vi "UHR-Fleezers Control (host) -TL - oscillation.vi"(0 "Tab Control":T5(tab)) -> ()   [LabVIEW 2013] (continued)
    n1506 = Split 1D Array(array=w2057, index="N El. to Ave.") -> (second subarray=w2060:dbl[])  [unwired: 1 out]
    n1507 = Split 1D Array(array=w2054, index="N El. to Ave.") -> (second subarray=w2059:dbl[])  [unwired: 1 out]
    n1508 = local read "Trap X AI1 (DMA)"() -> (w2058:T13)
    n1509 = Multiply(x=w2132, y="Trap Disp. Downsample") -> (x*y=w2071:dbl)
    "Display Period (s)" <- w2071
    n1510 = Bundle("BD 1 Frequency 1 (MHz)"=w2026, "BD 1 Frequency 2 (MHz)"=w2025) -> (w2027:T45)  [unwired: 1 out]
    n1511 = for "Trap AI" {
      tunnel: [w2677] -> w2257 mode=indexing
      tunnel: w2069 -> [w2667]
      tunnel: "Trap Disp. Downsample" -> [w2675]
      tunnel: w2150 -> [w2673] mode=indexing
      tunnel: w2132 -> [w2672]
      tunnel: w2149 -> [w2671] mode=indexing
      tunnel: w2068 -> [w2670]
      tunnel: [w2669] -> w2107 mode=indexing
      tunnel: w2071 -> [w2668]
      n1512 = Bundle By Name("Y"=w2673, "dt"=w2672) -> (w2674:waveform(dbl))  [unwired: 1 out]
      n1513 = Set Waveform Attribute(5:w2671, 6:w2670, 7:w2674) -> (3:w2669:waveform(dbl))  [unwired: 1 in, 2 out]
      n1514 = call "downsample 1D array - double.vi"("Ave N"=w2675, "Array In"=w2673) -> ("Array Out"=w2676:dbl[])  [unwired: 1 out]
      n1515 = Bundle By Name(cluster=w2669, "t0"=w2667, "Y"=w2676, "dt"=w2668) -> (w2677:waveform(dbl))
    }
    n1516 = call-poly <vilib>:"Mean.vi"("X"=w2059) -> ("mean"=w2047:dbl)  [unwired: 1 out]
    n1517 = call-poly <vilib>:"Mean.vi"("X"=w2060) -> ("mean"=w2048:dbl)  [unwired: 1 out]
    n1518 = Cluster To Array(cluster=w2027) -> (array=w2024:dbl[])
    n1519 = Reciprocal(x=w2071) -> (1/x=→"Trap Disp. Freq. (Hz)":dbl)
    n1520 = local read "Data points/scans (MCL)"() -> (w2237:dbl)
    n1521 = To Fixed-Point(number=w2047) -> (fixed-point=w2045:fxp<+/-,16,1>)  [unwired: 1 in]
    n1522 = To Fixed-Point(number=w2048) -> (fixed-point=w2046:fxp<+/-,16,1>)  [unwired: 1 in]
    n1523 = Bundle("Trap 1 Pos.", "Trap 2 Pos.") -> (w2067:cluster{string, string})  [unwired: 1 out]
    n1524 = Bundle By Name(cluster=w2058, "Set 1"=w2046, "Set 2"=w2045) -> (→"Trap X AI1 (DMA)":T13)
    n1525 = Cluster To Array(cluster=w2067) -> (array=w2064:string[])
    n1526 = for "Trap Position" {
      tunnel: w2073 -> [w2317] mode=indexing
      tunnel: "Trap Disp. Downsample" -> [w2316]
      tunnel: w2071 -> [w2314]
      tunnel: w2069 -> [w2313]
      tunnel: w2068 -> [w2311]
      tunnel: w2064 -> [w2310] mode=indexing
      tunnel: [w2309] -> w2022 mode=indexing
      tunnel: w2024 -> [w2307] mode=indexing
      tunnel: w2023 -> [w2305]
      n1527 = call "downsample 1D array - double.vi"("Ave N"=w2316, "Array In"=w2317) -> ("Array Out"=w2315:dbl[])  [unwired: 1 out]
      n1528 = Subtract(x=w2315, y=w2307) -> (x-y=w2308:dbl[])
      n1529 = Multiply(x=w2305, y=w2308) -> (x*y=w2306:dbl[])
      n1530 = Bundle By Name("Y"=w2306, "dt"=w2314, "t0"=w2313) -> (w2312:waveform(dbl))  [unwired: 1 out]
      n1531 = Set Waveform Attribute(5:w2310, 6:w2311, 7:w2312) -> (3:w2309:waveform(dbl))  [unwired: 1 in, 2 out]
    }
    "Trap Positions" <- w2022
    n1532 = Bundle("APD 1", "APD 2") -> (w2256:cluster{string, string})  [unwired: 1 out]
    n1533 = Cluster To Array(cluster=w2256) -> (array=w2253:string[])
    n1534 = for "APD" {
      tunnel: w2226 -> [w2656] mode=indexing
      tunnel: w2096 -> [w2664]
      tunnel: [w2660] -> w2103 mode=indexing
      tunnel: "APD Disp. Scale" -> [w2661]
      tunnel: w2068 -> [w2659]
      tunnel: w2253 -> [w2658] mode=indexing
      tunnel: "APD Disp. Downsample" -> [w2654]
      tunnel: [w2657] -> w2252
      tunnel: w2069 -> [w2653]
      n1535 = call "integrate 1D array interval - double.vi"("Ave N"=w2654, "Array In"=w2656) -> ("Array Out"=w2655:dbl[])  [unwired: 1 out]
      n1536 = Multiply(x=w2664, y=w2654) -> (x*y=w2657:dbl)
      n1537 = Divide(x=w2655, y=w2661) -> (x/y=w2662:dbl[])
      n1538 = Bundle By Name("t0"=w2653, "Y"=w2662, "dt"=w2657) -> (w2663:waveform(dbl))  [unwired: 1 out]
      n1539 = Set Waveform Attribute(5:w2658, 6:w2659, 7:w2663) -> (3:w2660:waveform(dbl))  [unwired: 1 in, 2 out]
    }
    "APD Display Period (s)" <- w2252
    n1540 = Reciprocal(x=w2252) -> (1/x=→"APD Display Freq. (Hz)":dbl)
    n1541 = local read "Display Period (s)"() -> (w2131:dbl)
    n1542 = Increment(x=w2237) -> (x+1=w2238:dbl)
    n1543 = Index Array(array=w2022, index=0) -> (element=w2020:waveform(dbl))
    n1544 = To Double Precision Float(number=w2147) -> (double precision float=w2146:dbl[])
    n1545 = feedback #2(w2238) -> (w2241:dbl)
    n1546 = Select(t=0, s=w2228, f=w2241) -> (s? t:f=w2234:dbl)
    n1547 = Array Size(array=w2146) -> (size(s)=w2240:i32)
    n1548 = Add(x=w2240, y=w2234) -> (x+y=w2235:dbl)
    n1549 = Unbundle By Name(w2020) -> ("Y"=w2018:dbl[])
    n1550 = feedback #3(w2147) -> (w2224:u32[])
    n1551 = Build Array (concatenate)(w2224, w2147) -> (w2221:u32[])
    n1552 = feedback #4(w2083) -> (w2102:u32[])
    n1553 = Divide(x="Bead Sep. Int. Time (s)", y=w2131) -> (x/y=w2016:dbl)
    n1554 = Build Array (concatenate)(w2102, w2083) -> (w2101:u32[])
    n1555 = Greater?(x=w2235, y=w2237) -> (0:w2236:bool)
    n1556 = feedback #5(w2018) -> (w2019:dbl[])
    n1557 = Build Array (concatenate)(w2018, w2019) -> (w2017:dbl[])
    n1558 = Select(t=w2234, s=w2236, f=w2235) -> (s? t:f=w2233:dbl)
    n1559 = feedback-in #2(w2233) -> ()
    n1560 = Array Size(array=w2221) -> (size(s)=w2218:i32)
    n1561 = Array Size(array=w2147) -> (size(s)=w2220:i32)
    n1562 = local read "MCL Scanning"() -> (w2231:bool)
    n1563 = local read "APD Integration Time (s)"() -> (w2110:dbl)
    n1564 = Build Array (concatenate)(w2103, w2257) -> (w2105:waveform(dbl)[])
    "All Signals" <- w2105
    n1565 = Split 1D Array(array=w2017, index=w2016) -> (first subarray=w2010:dbl[])  [unwired: 1 out]
    n1566 = feedback-in #5(w2010) -> ()
    n1567 = Multiply(x=w2220, y="APD Ave N") -> (x*y=w2219:dbl)
    n1568 = Greater?(x=w2218, y=w2219) -> (0:w2222:bool)
    n1569 = Not(x=w2236) -> (.not. x?=w2230:bool)
    n1570 = To Double Precision Float(number=w2083) -> (double precision float=w2082:dbl[])
    n1571 = call-poly <vilib>:"Mean.vi"("X"=w2010) -> ("mean"=w2009:dbl)  [unwired: 1 out]
    "Mean T1 Position (nm)" <- w2009
    n1572 = Subtract(x=w2010, y=w2009) -> (x-y=w2015:dbl[])
    n1573 = Square(x=w2015) -> (x^2=w2014:dbl[])
    n1574 = And(x=w2230, y=w2231) -> (x .and. y?=w2232:bool)
    n1575 = call-poly <vilib>:"Mean.vi"("X"=w2014) -> ("mean"=w2013:dbl)  [unwired: 1 out]
    n1576 = case shown="True" w2222 {
      tunnel: w2221 -> [w2437 w2444]
      tunnel: [w2437 w2442] -> w2163
      tunnel: w2219 -> [_ w2439]
      tunnel: w2218 -> [_ w2443]
      tunnel: w2101 -> [w2436 w2441]
      tunnel: [w2436 w2438] -> w2098
      frame False {
      }
      frame True {
        n1577 = Subtract(x=w2443, y=w2439) -> (x-y=w2440:dbl)
        n1578 = Array Subset(array=w2444, index=w2440, length=w2439) -> (w2442:u32[])
        n1579 = Array Subset(array=w2441, index=w2440, length=w2439) -> (w2438:u32[])
      }
    }
    n1580 = feedback-in #3(w2163) -> ()
    n1581 = feedback-in #4(w2098) -> ()
    n1582 = Or(x=w2232, y=w2228) -> (x .or. y?=w2229:bool)
    n1583 = Square Root(x=w2013) -> (sqrt(x)=w2012:dbl)
    n1584 = Equal?(x="Tab Control 6", y=T35."High Res Display") -> (x = y?=w2153:bool)
    n1585 = Multiply(x="APD Disp. Scale", y=w2103) -> (x*y=w2112:waveform(dbl)[])
    n1586 = Multiply(x="APD Disp. Downsample", y=w2110) -> (x*y=w2108:dbl)
    n1587 = Multiply(x=10.0, y=w2012) -> (x*y=→"Trap 1 Position RMS (A)":dbl)
    n1588 = Divide(x=w2112, y=w2108) -> (x/y=w2080:waveform(dbl)[])
    n1589 = Index Array(array=w2080, index=0) -> (element=w2090:waveform(dbl))
    n1590 = case "For computing FFTs for display" shown="True" "Compute FFT" {
      tunnel: w2107 -> [_ w3114]
      frame False {
      }
      frame True {
        n1591 = Build Array("FFT 1 Choice 1", "FFT 1 Choice 2", "FFT 2 Choice 1", "FFT 2 Choice 2") -> (w3107:u16[])
        n1592 = Array Size(array=w3114) -> (size(s)=w3113:i32)
        n1593 = feedback-in #6(w3107) -> ()
        n1594 = feedback #6(u16[] [100, 100, 100, 100]) -> (w3108:u16[])
        n1595 = feedback-in #7("# Spectra to Ave.") -> ()
        n1596 = feedback #7("# Spectra to Ave.") -> (w3105:dbl)
        n1597 = Not Equal?(x="# Spectra to Ave.", y=w3105) -> (x != y?=w3104:bool)
        n1598 = Not Equal?(x=w3107, y=w3108) -> (x != y?=w3106:bool)
        n1599 = feedback #8(1.0) -> (w3091:dbl)
        n1600 = Compound Arithmetic op=OR("Reset FFT", w3106, w3104) -> (w3089:bool)
        n1601 = Select(t=1.0, s=w3089, f=w3091) -> (s? t:f=w3093:dbl)
        n1602 = Greater?(x=w3093, y="# Spectra to Ave.") -> (0:w3112:bool)
        n1603 = Increment(x=w3093) -> (x+1=w3092:dbl)
        n1604 = feedback-in #8(w3092) -> ()
        n1605 = local read "DMA Update Period (s)"() -> (w3087:dbl)
        n1606 = Multiply(x="# Spectra to Ave.", y=w3087) -> (x*y=→"Ave. Time (s)":dbl)
        n1607 = Build Array(cluster{"f0":dbl, "df":dbl, "magnitude":dbl[]} {"f0"=0.0, "df"=0.0, "magnitude"=[]} ("PSD")) -> (w3096:cluster{"f0":dbl, "df":dbl, "magnitude":dbl[]}[])
        n1608 = Build Array(w3096, w3096, w3096, w3096) -> (w3098:T46)
        n1609 = feedback #9(w3098) -> (w3103:T46)
        n1610 = for {
          N: 4 -> [_]
          tunnel: w3107 -> [w3136] mode=indexing
          tunnel: w3114 -> [w3137]
          tunnel: w3113 -> [w3139]
          tunnel: w3089 -> [w3132]
          tunnel: w3112 -> [w3131]
          tunnel: "# Spectra to Ave." -> [w3130]
          tunnel: [w3129] -> w3102 mode=indexing
          tunnel: w3103 -> [w3134] mode=indexing
          tunnel: [w3133] -> w3090 mode=indexing
          tunnel: w3093 -> [w3128]
          n1611 = Less?(x=w3136, y=w3139) -> (x < y?=w3138:bool)
          n1612 = Index Array(array=w3137, index=w3136) -> (element=w3135:waveform(dbl))
          n1613 = case shown="True" w3138 {
            tunnel: w3135 -> [_ w3156]
            tunnel: w3134 -> [w3141 w3154]
            tunnel: [w3141 w3142] -> w3133
            tunnel: w3132 -> [_ w3153]
            tunnel: w3131 -> [_ w3146]
            tunnel: w3130 -> [_ w3145]
            tunnel: [cluster{"f0":dbl, "df":dbl, "magnitude":dbl[]} {"f0"=0.0, "df"=0.0, "magnitude"=[]} ("PSD") w3147] -> w3129
            tunnel: w3128 -> [_ w3144]
            frame False {
            }
            frame True {
              n1614 = call <vilib>:"Std Deviation and Variance.vi"("X"=w3156) -> ("mean"=w3157:dbl)  [unwired: 1 in, 2 out]
              n1615 = Subtract(x=w3156, y=w3157) -> (x-y=w3155:waveform(dbl))
              n1616 = xnode "Spectral Measurements"("Signals"=w3155) -> ("PSD"=w3149:cluster{"f0":dbl, "df":dbl, "magnitude":dbl[]})  [unwired: 1 in, 1 out]
              n1617 = case shown="False" w3153 {
                tunnel: w3154 -> [w3166 _]
                tunnel: [w3162 w3171] -> w3142
                tunnel: w3149 -> [w3165 w3172]
                tunnel: w3146 -> [w3164 _]
                frame False {
                  n1618 = Build Array (concatenate)(w3166, w3165) -> (w3163:cluster{"f0":dbl, "df":dbl, "magnitude":dbl[]}[])
                  n1619 = case shown="True" w3164 {
                    tunnel: w3163 -> [w3167 w3170]
                    tunnel: [w3167 w3168] -> w3162
                    frame False {
                    }
                    frame True {
                      n1620 = Delete From Array(array=w3170, index=0) -> (array with subset deleted=w3168:cluster{"f0":dbl, "df":dbl, "magnitude":dbl[]}[])  [unwired: 1 in, 1 out]
                    }
                  }
                }
                frame True {
                  n1621 = Build Array(w3172) -> (w3171:cluster{"f0":dbl, "df":dbl, "magnitude":dbl[]}[])
                }
              }
              n1622 = for {
                tunnel: w3142 -> [w3161] mode=indexing
                tunnel: [w3160] -> w3152 mode=indexing
                workers-P: _ -> [_]
                n1623 = Unbundle By Name(w3161) -> ("magnitude"=w3160:dbl[])
              }
              n1624 = Transpose 2D Array(2D array=w3152) -> (transposed array=w3151:dbl[][])
              n1625 = for {
                tunnel: w3151 -> [w3159] mode=indexing
                tunnel: [w3158] -> w3150 mode=indexing
                workers-P: _ -> [_]
                n1626 = Add Array Elements(numeric array=w3159) -> (sum=w3158:dbl)
              }
              n1627 = Select(t=w3145, s=w3146, f=w3144) -> (s? t:f=w3143:dbl)
              n1628 = Divide(x=w3150, y=w3143) -> (x/y=w3148:dbl[])
              n1629 = Bundle By Name(cluster=w3149, "magnitude"=w3148) -> (w3147:cluster{"f0":dbl, "df":dbl, "magnitude":dbl[]})
            }
          }
        }
        n1630 = case shown="True" w3089 {
          tunnel: w3090 -> [w3121 w3127]
          tunnel: [w3121 w3122] -> w3088
          frame False {
          }
          frame True {
            n1631 = Array Subset(array=w3127, index (row)=0 ("index"), length (row)=4 ("length"), index (col)=0 ("index"), length (col)=1 ("length")) -> (w3122:T46)
          }
        }
        n1632 = feedback-in #9(w3088) -> ()
        n1633 = Split 1D Array(array=w3102, index=2) -> (first subarray=→"FFT 1":cluster{"f0":dbl, "df":dbl, "magnitude":dbl[]}[], second subarray=→"FFT 2":cluster{"f0":dbl, "df":dbl, "magnitude":dbl[]}[])
      }
    }
    n1634 = Index Array(array=w2080, index=1) -> (element=w2088:waveform(dbl))
    n1635 = case "For displaying the high resolution display (no downsampling)" shown="True" w2153 {
      tunnel: w2107 -> [_ w2337]
      frame False {
      }
      frame True {
        n1636 = Index Array(array=w2337, index="High Res. Display") -> (element=w2338:waveform(dbl))
        n1637 = call <vilib>:"Std Deviation and Variance.vi"("X"=w2338) -> ("mean"=w2345:dbl, "standard deviation"=w2350:dbl)  [unwired: 1 in, 1 out]
        "Mean Intensity" <- w2345
        "Sigma" <- w2350
        n1638 = Subtract(x=w2338, y=w2345) -> (x-y=w2344:waveform(dbl))
        n1639 = Select(t=w2344, s="Subtract mean", f=w2338) -> (s? t:f=→"1 Channel":waveform(dbl))
        n1640 = Divide(x=w2350, y=w2345) -> (x/y=→"Sigma/Mean":dbl)
        n1641 = feedback #10(1) -> (w2339:i32)
        n1642 = Greater Or Equal?(x=w2339, y="Slow mean N ave.") -> (x >= y?=w2352:bool)
        n1643 = Increment(x=w2339) -> (x+1=w2354:i32)
        n1644 = Select(t=1, s=w2352, f=w2354) -> (s? t:f=w2341:i32)
        n1645 = feedback-in #10(w2341) -> ()
        n1646 = feedback #11() -> (w2342:waveform(dbl))  [unwired: 1 out]
        n1647 = case shown="Default" w2339 {
          tunnel: [w2357 w2360] -> w2343
          tunnel: w2342 -> [w2359 _]
          tunnel: w2338 -> [w2358 w2360]
          frame Default {
            n1648 = call-poly <vilib>:"Append Waveforms.vi"("waveform B"=w2358, "waveform A"=w2359) -> ("waveform out"=w2357:waveform(dbl))  [unwired: 1 in, 8 out]
          }
          frame 1 {
          }
        }
        n1649 = feedback-in #11(w2343) -> ()
        n1650 = case shown="True" w2352 {
          tunnel: w2343 -> [_ w2356]
          frame False {
          }
          frame True {
            n1651 = call-poly <vilib>:"Mean.vi"("X"=w2356) -> ("mean"=→"Slow mean":dbl)  [unwired: 1 out]
          }
        }
      }
    }
    n1652 = case "For plotting results of scanning MCL" shown="True" w2229 {
      tunnel: w2228 -> [_ w2477]
      tunnel: w2146 -> [_ w2573]
      tunnel: w2237 -> [_ _]
      tunnel: w2107 -> [_ w2547]
      tunnel: w2082 -> [_ w2478]
      tunnel: w2081 -> [_ w2451]
      frame False {
      }
      frame True {
        w2458 = u32 0 items=["Horizontal", "Vertical", "Central", "1st Diagonal", "2nd Diagonal"] ("Type of Symmetry")
        w2486 = u32 0 items=["Horizontal", "Vertical", "Central", "1st Diagonal", "2nd Diagonal"] ("Type of Symmetry")
        w2489 = u32 0 items=["Horizontal", "Vertical", "Central", "1st Diagonal", "2nd Diagonal"] ("Type of Symmetry")
        w2518 = u32 0 items=["Horizontal", "Vertical", "Central", "1st Diagonal", "2nd Diagonal"] ("Type of Symmetry")
        n1653 = Index Array(array=w2547, index=10) -> (element=w2553:waveform(dbl))
        n1654 = Index Array(array=w2547, index=11) -> (element=w2550:waveform(dbl))
        n1655 = local read "Cycles/step (MCL)"() -> (w2503:u64)
        n1656 = Index Array(array=w2547, index="Channel") -> (element=w2549:waveform(dbl))
        n1657 = Unbundle(w2451) -> ("New Image"=w2450:T3, "New Image"=w2449:T3, "New Image"=w2448:T3, "New Image"=w2447:T3)
        n1658 = Unbundle By Name(w2553) -> ("Y"=w2505:dbl[])
        n1659 = Unbundle By Name(w2550) -> ("Y"=w2507:dbl[])
        n1660 = Unbundle By Name(w2549) -> ("Y"=w2512:dbl[])
        n1661 = call "downsample 1D array - double.vi"("Ave N"=w2503, "Array In"=w2505) -> ("Array Out"=w2504:dbl[])  [unwired: 1 out]
        n1662 = call "downsample 1D array - double.vi"("Ave N"=w2503, "Array In"=w2507) -> ("Array Out"=w2506:dbl[])  [unwired: 1 out]
        n1663 = call "downsample 1D array - double.vi"("Ave N"=w2503, "Array In"=w2512) -> ("Array Out"=w2511:dbl[])  [unwired: 1 out]
        n1664 = feedback #12(w2573) -> (w2574:dbl[])
        n1665 = Build Array (concatenate)(w2574, w2573) -> (w2555:dbl[])
        n1666 = feedback #13(w2478) -> (w2480:dbl[])
        n1667 = Build Array (concatenate)(w2480, w2478) -> (w2479:dbl[])
        n1668 = local read "Scan steps (MCL)"() -> (w2460:u64)
        n1669 = Select(t=w2573, s=w2477, f=w2555) -> (s? t:f=w2559:dbl[])
        n1670 = feedback-in #12(w2559) -> ()
        n1671 = Select(t=w2478, s=w2477, f=w2479) -> (s? t:f=w2461:dbl[])
        n1672 = feedback-in #13(w2461) -> ()
        n1673 = local read "Scan lines (y)"() -> (w2446:u64)
        n1674 = local read "N APD Samp/step"() -> (w2462:dbl)
        n1675 = feedback #14(w2504) -> (w2561:dbl[])
        n1676 = Build Array (concatenate)(w2561, w2504) -> (w2552:dbl[])
        n1677 = feedback #15(w2511) -> (w2571:dbl[])
        n1678 = Build Array (concatenate)(w2571, w2511) -> (w2570:dbl[])
        n1679 = feedback #16(w2506) -> (w2563:dbl[])
        n1680 = Build Array (concatenate)(w2563, w2506) -> (w2564:dbl[])
        n1681 = Select(t=w2504, s=w2477, f=w2552) -> (s? t:f=w2508:dbl[])
        n1682 = feedback-in #14(w2508) -> ()
        n1683 = Select(t=w2511, s=w2477, f=w2570) -> (s? t:f=w2510:dbl[])
        n1684 = feedback-in #15(w2510) -> ()
        n1685 = Select(t=w2506, s=w2477, f=w2564) -> (s? t:f=w2509:dbl[])
        n1686 = feedback-in #16(w2509) -> ()
        n1687 = Multiply(x=w2460, y=u64 2) -> (x*y=w2445:u64)
        n1688 = call "integrate 1D array interval - double.vi"("Ave N"=w2462, "Array In"=w2461) -> ("Array Out"=w2473:dbl[])  [unwired: 1 out]
        n1689 = call "integrate 1D array interval - double.vi"("Ave N"=w2462, "Array In"=w2559) -> ("Array Out"=w2558:dbl[])  [unwired: 1 out]
        n1690 = Array Size(array=w2473) -> (size(s)=w2474:i32)
        n1691 = Array Size(array=w2558) -> (size(s)=w2560:i32)
        n1692 = Multiply(x=w2446, y=w2445) -> (x*y=w2476:u64)
        n1693 = Multiply(x=w2446, y=w2445) -> (x*y=w2568:u64)
        n1694 = call-poly <vilib>:"Mean.vi"("X"=w2508) -> ("mean"=w2492:dbl)  [unwired: 1 out]
        n1695 = Subtract(x=w2476, y=w2474) -> (x-y=w2467:u64)
        n1696 = call-poly <vilib>:"Mean.vi"("X"=w2510) -> ("mean"=w2497:dbl)  [unwired: 1 out]
        n1697 = call-poly <vilib>:"Mean.vi"("X"=w2509) -> ("mean"=w2495:dbl)  [unwired: 1 out]
        n1698 = call-poly <vilib>:"Mean.vi"("X"=w2473) -> ("mean"=w2464:dbl)  [unwired: 1 out]
        n1699 = Subtract(x=w2568, y=w2560) -> (x-y=w2502:u64)
        n1700 = call-poly <vilib>:"Mean.vi"("X"=w2558) -> ("mean"=w2499:dbl)  [unwired: 1 out]
        n1701 = Initialize Array(1.0 ("element"), w2467) -> (w2463:dbl[])
        n1702 = Initialize Array(1.0 ("element"), w2502) -> (w2493:dbl[])
        n1703 = Multiply(x=w2463, y=w2464) -> (x*y=w2465:dbl[])
        n1704 = Multiply(x=w2493, y=w2495) -> (x*y=w2496:dbl[])
        n1705 = Multiply(x=w2493, y=w2497) -> (x*y=w2498:dbl[])
        n1706 = Multiply(x=w2493, y=w2492) -> (x*y=w2494:dbl[])
        n1707 = Multiply(x=w2493, y=w2499) -> (x*y=w2500:dbl[])
        n1708 = Build Array (concatenate)(w2508, w2494) -> (w2562:dbl[])
        n1709 = Build Array (concatenate)(w2510, w2498) -> (w2566:dbl[])
        n1710 = Build Array (concatenate)(w2509, w2496) -> (w2565:dbl[])
        n1711 = Build Array (concatenate)(w2473, w2465) -> (w2475:dbl[])
        n1712 = Build Array (concatenate)(w2558, w2500) -> (w2567:dbl[])
        n1713 = Reshape Array(w2562, w2446, w2445) -> (w2528:dbl[][])
        n1714 = Reshape Array(w2475, w2446, w2445) -> (w2471:dbl[][])
        n1715 = Reshape Array(w2566, w2446, w2445) -> (w2520:dbl[][])
        n1716 = Reshape Array(w2565, w2446, w2445) -> (w2535:dbl[][])
        n1717 = Reshape Array(w2567, w2446, w2445) -> (w2545:dbl[][])
        n1718 = Array Subset(array=w2535, index (col)=0 ("index"), length (col)=w2460) -> (w2540:dbl[][])  [unwired: 2 in]
        n1719 = Array Subset(array=w2535, index (col)=w2460) -> (w2538:dbl[][])  [unwired: 3 in]
        n1720 = Array Subset(array=w2520, index (col)=0 ("index"), length (col)=w2460) -> (w2526:dbl[][])  [unwired: 2 in]
        n1721 = Array Subset(array=w2520, index (col)=w2460) -> (w2524:dbl[][])  [unwired: 3 in]
        n1722 = Array Subset(array=w2471, index (col)=0 ("index"), length (col)=w2460) -> (w2470:dbl[][])  [unwired: 2 in]
        n1723 = Array Subset(array=w2471, index (col)=w2460) -> (w2468:dbl[][])  [unwired: 3 in]
        n1724 = Array Subset(array=w2545, index (col)=0 ("index"), length (col)=w2460) -> (w2544:dbl[][])  [unwired: 2 in]
        n1725 = Array Subset(array=w2545, index (col)=w2460) -> (w2542:dbl[][])  [unwired: 3 in]
        n1726 = Array Subset(array=w2528, index (col)=0 ("index"), length (col)=w2460) -> (w2533:dbl[][])  [unwired: 2 in]
        n1727 = Array Subset(array=w2528, index (col)=w2460) -> (w2531:dbl[][])  [unwired: 3 in]
        n1728 = for {
          tunnel: w2540 -> [w2582] mode=indexing
          tunnel: [w2581] -> w2539 mode=indexing
          workers-P: _ -> [_]
          n1729 = Reverse 1D Array(array=w2582) -> (reversed array=w2581:dbl[])
        }
        n1730 = for {
          tunnel: w2526 -> [w2578] mode=indexing
          tunnel: [w2577] -> w2525 mode=indexing
          workers-P: _ -> [_]
          n1731 = Reverse 1D Array(array=w2578) -> (reversed array=w2577:dbl[])
        }
        n1732 = for {
          tunnel: w2470 -> [w2576] mode=indexing
          tunnel: [w2575] -> w2469 mode=indexing
          workers-P: _ -> [_]
          n1733 = Reverse 1D Array(array=w2576) -> (reversed array=w2575:dbl[])
        }
        n1734 = for {
          tunnel: w2544 -> [w2584] mode=indexing
          tunnel: [w2583] -> w2543 mode=indexing
          workers-P: _ -> [_]
          n1735 = Reverse 1D Array(array=w2584) -> (reversed array=w2583:dbl[])
        }
        n1736 = for {
          tunnel: w2533 -> [w2580] mode=indexing
          tunnel: [w2579] -> w2532 mode=indexing
          workers-P: _ -> [_]
          n1737 = Reverse 1D Array(array=w2580) -> (reversed array=w2579:dbl[])
        }
        n1738 = Index Array(array=w2545, index (row)=0) -> (element=→"Waveform Graph":dbl[])  [unwired: 1 in]
        n1739 = Add(x=w2539, y=w2538) -> (x+y=w2537:dbl[][])
        n1740 = Add(x=w2525, y=w2524) -> (x+y=w2523:dbl[][])
        n1741 = Add(x=w2469, y=w2468) -> (x+y=w2453:dbl[][])
        n1742 = Add(x=w2543, y=w2542) -> (x+y=w2517:dbl[][])
        n1743 = Add(x=w2532, y=w2531) -> (x+y=w2530:dbl[][])
        n1744 = Divide(x=w2523, y=2) -> (x/y=w2521:dbl[][])
        n1745 = Divide(x=w2537, y=2) -> (x/y=w2482:dbl[][])
        n1746 = Divide(x=w2530, y=2) -> (x/y=w2484:dbl[][])
        n1747 = To Single Precision Float(number=w2517) -> (single precision float=w2516:sgl[][])
        n1748 = Transpose 2D Array(2D array=w2521) -> (transposed array=→"Data map":dbl[][])
        n1749 = To Single Precision Float(number=w2453) -> (single precision float=w2457:sgl[][])
        n1750 = To Single Precision Float(number=w2482) -> (single precision float=w2488:sgl[][])
        n1751 = To Single Precision Float(number=w2484) -> (single precision float=w2485:sgl[][])
        n1752 = call "IMAQ ArrayToImage"("Image Pixels (Float)"=w2516, "Image"=w2450) -> ("Image Out"=w2519:T3)  [unwired: 8 in, 1 out]
        n1753 = call "IMAQ ArrayToImage"("Image Pixels (Float)"=w2457, "Image"=w2449) -> ("Image Out"=w2459:T3)  [unwired: 8 in, 1 out]
        n1754 = call "IMAQ ArrayToImage"("Image Pixels (Float)"=w2488, "Image"=w2448) -> ("Image Out"=w2490:T3)  [unwired: 8 in, 1 out]
        n1755 = call "IMAQ ArrayToImage"("Image Pixels (Float)"=w2485, "Image"=w2447) -> ("Image Out"=w2487:T3)  [unwired: 8 in, 1 out]
        n1756 = call "IMAQ Symmetry"("Type of Symmetry"=w2518, "Image Src"=w2519) -> ("Image Dst Out"=w2514:T3)  [unwired: 3 in, 1 out]
        n1757 = call "IMAQ Symmetry"("Type of Symmetry"=w2458, "Image Src"=w2459) -> ("Image Dst Out"=w2455:T3)  [unwired: 3 in, 1 out]
        n1758 = call "IMAQ Symmetry"("Type of Symmetry"=w2489, "Image Src"=w2490) -> ("Image Dst Out"=→"Detection Laser X":T3)  [unwired: 3 in, 1 out]
        n1759 = call "IMAQ Symmetry"("Type of Symmetry"=w2486, "Image Src"=w2487) -> ("Image Dst Out"=→"Detection Laser Y":T3)  [unwired: 3 in, 1 out]
        n1760 = call "IMAQ Set Simple Calibration"("Calibration Axis Info"=T36 {"Origin Pixel"={"X"=0.0, "Y"=0.0}, "Angle Relative to Horizontal (deg)"=0.0, "Axis Reference"=0}, "Grid Descriptor"=T37 {"X Step"=0.3, "Y Step"=0.3, "Unit"=enum."Undefined"}, "Image"=w2514) -> ("Calibrated Image"=→"APD 1":T3)  [unwired: 7 in, 1 out]
        n1761 = call "IMAQ Set Simple Calibration"("Calibration Axis Info"=T36 {"Origin Pixel"={"X"=0.0, "Y"=0.0}, "Angle Relative to Horizontal (deg)"=0.0, "Axis Reference"=0}, "Grid Descriptor"=T37 {"X Step"=0.3, "Y Step"=0.3, "Unit"=enum."Undefined"}, "Image"=w2455) -> ("Calibrated Image"=→"APD 2":T3)  [unwired: 7 in, 1 out]
      }
    }
    n1762 = Subtract(x=w2088, y="APD 2 Offset") -> (x-y=w2085:waveform(dbl))
    n1763 = Subtract(x=w2090, y="APD 1 Offset") -> (x-y=w2086:waveform(dbl))
    n1764 = Index Array(array=w2105, index=3) -> (element=w2173:waveform(dbl))
    n1765 = Index Array(array=w2105, index=6) -> (element=w2170:waveform(dbl))
    n1766 = Build Array(w2086, w2085) -> (→"APD Chart":waveform(dbl)[])
    n1767 = Array Size(array=w2163) -> (size(s)=w2217:i32)
    n1768 = call <vilib>:"Std Deviation and Variance.vi"("X"=w2098) -> ("standard deviation"=w2097:dbl)  [unwired: 1 in, 2 out]
    n1769 = Add Array Elements(numeric array=w2098) -> (sum=w2100:u32)
    n1770 = Add Array Elements(numeric array=w2163) -> (sum=w2227:u32)
    n1771 = call <vilib>:"Std Deviation and Variance.vi"("X"=w2163) -> ("standard deviation"=w2162:dbl)  [unwired: 1 in, 2 out]
    n1772 = Divide(x="T1 offset_x (mV)", y=1000.0) -> (x/y=w2174:dbl)
    n1773 = Divide(x=w2097, y=w2096) -> (x/y=w2093:dbl)
    "Rate sigma (Hz) 2" <- w2093
    n1774 = Multiply(x=w2096, y=w2217) -> (x*y=w2099:dbl)
    "Int. Time (s)" <- w2099
    n1775 = Divide(x=w2100, y=w2099) -> (x/y=w2094:dbl)
    "APD 2 Rate (Hz)" <- w2094
    n1776 = Divide(x=w2227, y=w2099) -> (x/y=w2160:dbl)
    "APD 1 Rate (Hz)" <- w2160
    n1777 = Divide(x=w2162, y=w2096) -> (x/y=w2161:dbl)
    "Rate sigma (Hz)" <- w2161
    n1778 = Divide(x=w2093, y=w2094) -> (x/y=→"Sigma/Mean 2":dbl)
    n1779 = Divide(x=w2161, y=w2160) -> (x/y=→"Sigma/Mean":dbl)
    n1780 = Divide(x="T2 offset_x (mV)", y=1000.0) -> (x/y=w2172:dbl)
    n1781 = case shown="1" "Calibration" {
      tunnel: "T1 alpha_x (nm/V)" -> [_ w2413 w2434]
      tunnel: "T1 kappa_x (pN/nm)" -> [_ _ w2424]
      tunnel: "T2 alpha_x (nm/V)" -> [_ w2412 w2432]
      tunnel: "T2 kappa_x (pN/nm)" -> [_ _ w2425]
      tunnel: w2173 -> [w2395 w2410 w2430]
      tunnel: w2170 -> [w2394 w2408 w2428]
      tunnel: [w2395 w2407 w2427] -> w2203
      tunnel: [w2394 w2406 w2426] -> w2202
      tunnel: ["T1 X (V)" ("Label.Text") "T1 X (nm)" ("Label.Text") "T1 X (pN)" ("Label.Text")] -> w2191
      tunnel: ["T2 X (V)" ("Label.Text") "T2 X (nm)" ("Label.Text") "T2 X (pN)" ("Label.Text")] -> w2190
      tunnel: ["Position (V)" ("Label.Text") "Position (nm)" ("Label.Text") "Force (pN)" ("Label.Text")] -> w2192
      tunnel: w2172 -> [_ w2398 w2417]
      tunnel: w2174 -> [_ w2401 w2419]
      tunnel: ["Mean (V)" ("Label.Text") "Mean (nm)" ("Label.Text") "Mean (pN)" ("Label.Text")] -> w2187
      tunnel: ["Difference (V)" ("Label.Text") "Difference (nm)" ("Label.Text") "Difference (pN)" ("Label.Text")] -> w2113
      frame 0, Default {
      }
      frame 1 {
        # "position"
        n1782 = Unbundle By Name(w2410) -> ("Y"=w2414:dbl[])
        n1783 = Unbundle By Name(w2408) -> ("Y"=w2399:dbl[])
        n1784 = Subtract(x=w2414, y=w2401) -> (x-y=w2402:dbl[])
        n1785 = Subtract(x=w2399, y=w2398) -> (x-y=w2400:dbl[])
        n1786 = Multiply(x=w2400, y=w2412) -> (x*y=w2409:dbl[])
        n1787 = Multiply(x=w2413, y=w2402) -> (x*y=w2411:dbl[])
        n1788 = Bundle By Name(cluster=w2408, "Y"=w2409) -> (w2406:waveform(dbl))
        n1789 = Bundle By Name(cluster=w2410, "Y"=w2411) -> (w2407:waveform(dbl))
      }
      frame 2 {
        # "force"
        n1790 = Unbundle By Name(w2430) -> ("Y"=w2435:dbl[])
        n1791 = Unbundle By Name(w2428) -> ("Y"=w2433:dbl[])
        n1792 = Subtract(x=w2433, y=w2417) -> (x-y=w2418:dbl[])
        n1793 = Subtract(x=w2435, y=w2419) -> (x-y=w2420:dbl[])
        n1794 = Compound Arithmetic op=MULTIPLY(w2418, w2432, w2425) -> (w2429:dbl[])
        n1795 = Compound Arithmetic op=MULTIPLY(w2424, w2434, w2420) -> (w2431:dbl[])
        n1796 = Bundle By Name(cluster=w2428, "Y"=w2429) -> (w2426:waveform(dbl))
        n1797 = Bundle By Name(cluster=w2430, "Y"=w2431) -> (w2427:waveform(dbl))
      }
    }
    n1798 = feedback-in #17("Calibration") -> ()
    n1799 = feedback #17(u16 1 ("Calibration")) -> (w2194:u16)
    n1800 = local read "Trap 2 Bead Size (nm)"() -> (w1992:dbl)
    n1801 = local read "Trap 1 Bead Size (nm)"() -> (w1991:dbl)
    n1802 = local read "AOM X Cal (nm/MHz)"() -> (w1989:dbl)
    n1803 = local read "Trap Delta (MHz)"() -> (w1988:dbl)
    n1804 = Not Equal?(x=w2194, y="Calibration") -> (x != y?=w2151:bool)
    n1805 = Multiply(x=w1989, y=w1988) -> (x*y=w1993:dbl)
    n1806 = Add(x=w1992, y=w1991) -> (x+y=w1995:dbl)
    n1807 = Unbundle By Name(w2173) -> ("Y"=w2176:dbl[])
    n1808 = Unbundle By Name(w2170) -> ("Y"=w2179:dbl[])
    n1809 = Divide(x=w1995, y=2.0) -> (x/y=w1990:dbl)
    n1810 = Subtract(x=w2176, y=w2174) -> (x-y=w2177:dbl[])
    n1811 = Subtract(x=w2179, y=w2172) -> (x-y=w2178:dbl[])
    n1812 = disable-structure shown="Enabled" {
      disable-tunnel: [-1.0 ("y") 1.0] -> w2180
      frame Disabled {
      }
      frame Enabled {
      }
    }
    n1813 = Multiply(x=w2178, y="T2 alpha_x (nm/V)") -> (x*y=w2169:dbl[])
    n1814 = Multiply(x="T1 alpha_x (nm/V)", y=w2177) -> (x*y=w2168:dbl[])
    n1815 = Multiply(x=w2202, y=w2180) -> (x*y=w2181:waveform(dbl))
    n1816 = case shown="False" "Read Lateness and Rel Phase" {
      tunnel: w2005 -> [w2361 w2383]
      tunnel: w2004 -> [w2362 w2382]
      tunnel: [w2361 w2381] -> w2166
      tunnel: [w2362 w2380] -> w2165
      frame False {
      }
      frame True {
        n1817 = xnode "Read/Write Control"("FPGA VI Reference In"=w2383, "error in"=w2382) -> ("FPGA VI Reference Out"=w2381:T19, "error out"=w2380:errorcluster, "GI Relative phase"=→"GI relative phase":i16, "Relative phase"=→"Relative phase (AI1)":i16, "AI Late Counter"=→"Late Counter (AI1)":u16, "GI Late Counter"=→"GI Late Counter":u16, "MCL Late Counter"=→"MCL Late Counter":u16, "MCL Relative Phase"=→"Relative Phase (MCL)":i16, "APD Acq Relative Phase"=→"APD Acq Relative Phase":i16, "APD 1 Gate Relative Phase"=→"APD 1 Gate Relative Phase":i16, "APD 2 Gate Relative Phase"=→"APD 2 Gate Relative Phase":i16, "APD Acq Late Counter"=→"APD Acq Late Counter":u16, "APD 1 Gate Late Counter"=→"APD 1 Gate Late Counter":u16, "APD 2 Gate Late Counter"=→"APD 2 Gate Late Counter":u16, "Green FB Relative Phase"=→"Relative phase (Green FB)":i16, "GI Relative phase 2"=→"GI relative phase 2":i16, "GI Late Counter 2"=→"GI Late Counter 2":u16, "Trap Pos FIFO Timeout"=→"Trap Pos FIFO Timeout":u16, "Trap AI FIFO Timeout"=→"Trap AI FIFO Timeout":u16)
      }
    }
    n1818 = Subtract(x=w2169, y=w2168) -> (x-y=w1987:dbl[])
    n1819 = call-poly <vilib>:"Mean.vi"("X"=w1987) -> ("mean"=w1994:dbl)  [unwired: 1 out]
    n1820 = Add(x=w1993, y=w1994) -> (x+y=w1997:dbl)
    n1821 = Subtract(x=w1997, y=w1990) -> (x-y=→"Tether Extension (nm, calculated)":dbl)
    n1822 = Unbundle By Name(w2202) -> ("Y"=w2138:dbl[])
    n1823 = Unbundle By Name(w2203) -> ("Y"=w2139:dbl[])
    n1824 = Build Array(w2203, w2181) -> (→"Force":waveform(dbl)[])
    n1825 = Subtract(x=w1987, y="Offset (nm)") -> (x-y=w2136:dbl[])
    n1826 = call-poly <vilib>:"Mean.vi"("X"=w2138) -> ("mean"=w2117:dbl)  [unwired: 1 out]
    "T2 X" <- w2117
    n1827 = Absolute Value(x=w2139) -> (abs(x)=w2140:dbl[])
    n1828 = Absolute Value(x=w2138) -> (abs(x)=w2141:dbl[])
    n1829 = call-poly <vilib>:"Mean.vi"("X"=w2139) -> ("mean"=w2118:dbl)  [unwired: 1 out]
    "T1 X" <- w2118
    n1830 = Add(x=w2140, y=w2141) -> (x+y=w2142:dbl[])
    n1831 = Bundle By Name(cluster=w2173, "Y"=w2136) -> (w2104:waveform(dbl))
    "Bead Separation" <- w2104
    n1832 = Divide(x=w2142, y=2.0) -> (x/y=→"Vec Mean of T1 T2":dbl[])
    n1833 = case shown="True" w2151 {
      tunnel: w2192 -> [_ w2388]
      tunnel: w2191 -> [_ w2387]
      tunnel: w2190 -> [_ w2386]
      tunnel: w2187 -> [_ w2385]
      tunnel: w2113 -> [_ w2384]
      frame False {
      }
      frame True {
        n1834 = property on="Force" class="WFChart (strict)"("YScale.NameLbl.Text"=w2388) -> ()  [unwired: 2 in, 2 out]
        n1835 = property on="T2 X" class="DigNum (strict)"("Caption.Text"=w2386) -> ()  [unwired: 2 in, 2 out]
        n1836 = property on="T1 X" class="DigNum (strict)"("Caption.Text"=w2387) -> ()  [unwired: 2 in, 2 out]
        n1837 = property on="Mean" class="DigNum (strict)"("Caption.Text"=w2385) -> ()  [unwired: 2 in, 2 out]
        n1838 = property on="Difference" class="DigNum (strict)"("Caption.Text"=w2384) -> ()  [unwired: 2 in, 2 out]
      }
    }
    n1839 = local read "Tether"() -> (w2145:bool)
    n1840 = Absolute Value(x=w2118) -> (abs(x)=w2115:dbl)
    n1841 = Absolute Value(x=w2117) -> (abs(x)=w2114:dbl)
    n1842 = Add(x=w2115, y=w2114) -> (x+y=w2189:dbl)
    n1843 = Subtract(x=w2115, y=w2114) -> (x-y=→"Difference":dbl)
    n1844 = feedback #18(w2136) -> (w2135:dbl[])
    n1845 = Divide(x=w2189, y=2.0) -> (x/y=w2144:dbl)
    "Mean" <- w2144
    n1846 = case shown="True" w2145 {
      tunnel: w2144 -> [_ w2320]
      frame False {
      }
      frame True {
        n1847 = Greater?(x="Lost Tether Alarm Threshold (pN)", y=w2320) -> (0:w2318:bool)
        n1848 = case shown="True" w2318 {
          frame False {
          }
          frame True {
            n1849 = flat-sequence {
              frame #0 {
                # "stop only if saving"
                n1850 = local read "Saving..."() -> (w2333:bool)
                n1851 = And(x=w2333, y="TA Cancel Save?") -> (x .and. y?=w2332:bool)
                n1852 = local write "Stop Saving"(w2332) -> ()
              }
              frame #1 {
                n1853 = case shown="True" "TA Green Off?" {
                  frame False {
                  }
                  frame True {
                    w2336 = FALSE ("Fl. Triggered...")
                    n1854 = local write "Fl. Triggered..."(w2336) -> ()
                    n1855 = property on="Green Laser ON/Interlacing" class="Bool (strict)"("Val(Sgnl)"=w2336) -> ()  [unwired: 2 in, 2 out]
                  }
                }
              }
            }
            n1856 = local read "Time tether formed"() -> (w2327:timestamp)
            n1857 = Get Date/Time In Seconds() -> (seconds since 1Jan1904=w2328:timestamp)
            n1858 = Subtract(x=w2328, y=w2327) -> (x-y=w2326:dbl)
            n1859 = Number To Decimal String(number=w2326) -> (decimal integer string=w2323:string)  [unwired: 1 out]
            n1860 = local read "Messages"() -> (w2330:string)
            n1861 = call <vilib>:"Beep.vi"() -> ()  [unwired: 3 in, 9 out]
            n1862 = Concatenate Strings("Lost tether (" ("Message to add"), w2323, " s)." ("string")) -> (w2325:string)
            n1863 = local write "Tether"(FALSE ("Tether")) -> ()
            n1864 = call "Update messages.vi"("Message to add"=w2325, "Old message string"=w2330) -> ("New message string"=w2329:string)
            n1865 = local write "Messages"(w2329) -> ()
            n1866 = property on="Trap Pos. FB ON" class="Bool (strict)"("Val(Sgnl)"=FALSE ("Value (Signaling)")) -> ()  [unwired: 2 in, 2 out]
          }
        }
      }
    }
    n1867 = Build Array (concatenate)(w2136, w2135) -> (w2134:dbl[])
    n1868 = Split 1D Array(array=w2134, index=w2016) -> (first subarray=w2130:dbl[])  [unwired: 1 out]
    n1869 = feedback-in #18(w2130) -> ()
    n1870 = call-poly <vilib>:"Mean.vi"("X"=w2130) -> ("mean"=w2129:dbl)  [unwired: 1 out]
    "Bead Mean (nm)" <- w2129
    n1871 = Subtract(x=w2130, y=w2129) -> (x-y=w2128:dbl[])
    n1872 = Square(x=w2128) -> (x^2=w2127:dbl[])
    n1873 = call-poly <vilib>:"Mean.vi"("X"=w2127) -> ("mean"=w2126:dbl)  [unwired: 1 out]
    n1874 = Square Root(x=w2126) -> (sqrt(x)=w2125:dbl)
    n1875 = Multiply(x=10.0, y=w2125) -> (x*y=→"RMS (Ang)":dbl)
    n1876 = xnode "Read/Write Control"("FPGA VI Reference In"=w2166, "error in"=w2165) -> ("FPGA VI Reference Out"=w2281:T19, "error out"=w2275:errorcluster, "AI2 Y Sum Set 1"=w2271:i16, "AI2 Y Sum Set 2"=w2270:i16, "AI1 X Set 1"=w2050:fxp<+/-,16,1>, "AI1 X Set 2"=w2049:fxp<+/-,16,1>, "Trap Pos FB Int Signal"=→"Trap Pos FB Int Signal":fxp<+/-,24,9>, "Trap Pos FB Int-Norm Signal"=→"Trap Pos FB Int-Norm Signal":fxp<+/-,16,1>, "Trap Pos FB Action"=w2043:i64, "Scanning"=→"AOD Scanning":bool, "Scan I"=→"AOD Scan I":u64, "Scanning MCL"=w2273:bool, "Scan I (MCL)"=→"MCL Scan I":u64, "Green FB Signals"=w2212:T47)  [unwired: 1 out]
    "MCL Scanning" <- w2273
    "Trap Pos FB Action" <- w2043
    n1877 = local read "AI2 (V)"() -> (w2272:cluster{"Set 1":dbl, "Set 2":dbl})
    n1878 = Bundle By Name(cluster=w2272, "Set 1"=w2271, "Set 2"=w2270) -> (w2268:cluster{"Set 1":dbl, "Set 2":dbl})
    n1879 = Divide(x=w2043, y=327.67) -> (x/y=→"Action (%)":dbl)
    n1880 = local read "Trap X (AI1)"() -> (w2063:T1)
    n1881 = Divide(x=w2268, y=3276.7) -> (x/y=w2267:cluster{"Set 1":dbl, "Set 2":dbl})
    n1882 = local write "AI2 (V)"(w2267) -> ()
    n1883 = Bundle(cluster=w2063, "Trap 1"=w2050, "Trap 2"=w2049) -> (→"Trap X (AI1)":T1)
    n1884 = Divide(x=w2212, y=3276.7) -> (x/y=w2208:T48)
    n1885 = Unbundle By Name(w2208) -> ("Green FB Ch 0"=w2211:dbl, "Green FB Ch 1"=w2210:dbl, "Green FB Ch 2"=w2209:dbl)
    n1886 = Divide(x=w2211, y=w2209) -> (x/y=w2207:dbl)
    n1887 = Divide(x=w2210, y=w2209) -> (x/y=w2206:dbl)
    n1888 = flat-sequence "To save data" {
      tunnel: [w3210] -> w2292
      tunnel: [w3211] -> w2291
      tunnel: w2243 -> [w3204]
      tunnel: w2132 -> [w3208]
      tunnel: ["Save Calibration"] -> w2264
      tunnel: w2261 -> [w3207]
      tunnel: [w3200] -> w2260
      tunnel: [w3197] -> w2259
      tunnel: [w3194] -> w2258
      tunnel: w2242 -> [w3196]
      tunnel: w2149 -> [w3190]
      tunnel: [w3190] -> w2148
      tunnel: ["Start Saving"] -> w2106
      tunnel: [w3184] -> w2032
      tunnel: [w3183] -> w2031
      tunnel: w2292 -> [w3445]
      tunnel: w2291 -> [w3444]
      tunnel: w2033 -> [w3443]
      tunnel: w2264 -> [w3442]
      tunnel: w2260 -> [w3440]
      tunnel: w2259 -> [w3439]
      tunnel: w2258 -> [w3438]
      tunnel: w2119 -> [w3437]
      tunnel: w2158 -> [w3436]
      tunnel: w2148 -> [w3435]
      tunnel: w2106 -> [w3434]
      tunnel: w2104 -> [w3433]
      tunnel: w2080 -> [w3432]
      tunnel: w2032 -> [w3431]
      tunnel: w2031 -> [w3430]
      tunnel: w2030 -> [w3429]
      frame #0 {
        n1889 = Or(x="Save N Sets", y="Start Saving") -> (x .or. y?=w3191:bool)
        n1890 = To Double Precision Float(number=w3207) -> (double precision float=w3201:dbl)
        n1891 = Build Array(w3191, "Save Calibration", w3204, w3196) -> (w3206:bool[])
        n1892 = Compound Arithmetic op=OR("Save Calibration", w3204, w3191, w3196) -> (w3209:bool)
        n1893 = Boolean Array To Number(Boolean array=w3206) -> (number=w3203:u32)
        n1894 = feedback #19(FALSE ("Save APD Data\nwith Trap Data")) -> (w3185:bool)
        n1895 = feedback #20(refnum<k0> refnum) -> (w3212:refnum<file>)
        n1896 = feedback #21(refnum<k0> refnum) -> (w3187:refnum<file>)
        n1897 = feedback #22(FALSE ("Save APD Data\nwith Trap Data")) -> (w3195:bool)
        n1898 = feedback #23(refnum<k0> refnum) -> (w3198:refnum<file>)
        n1899 = feedback #24(0) -> (w3214:i32)
        n1900 = feedback #25() -> (w3202:u32)  [unwired: 1 out]
        n1901 = case shown="True" w3209 {
          tunnel: [w3221 1] -> w3210
          tunnel: w3214 -> [w3223 _]
          tunnel: [w3222 w3241] -> w3211
          tunnel: w3212 -> [w3222 _]
          tunnel: w3208 -> [_ w3261]
          tunnel: w3201 -> [_ w3259]
          tunnel: w3203 -> [_ w3262]
          tunnel: [w3220 w3240] -> w3200
          tunnel: w3202 -> [w3220 _]
          tunnel: [w3219 w3238] -> w3197
          tunnel: w3198 -> [w3219 _]
          tunnel: [w3218 w3237] -> w3194
          tunnel: w3195 -> [w3218 _]
          tunnel: "Start Saving" -> [_ w3235]
          tunnel: w3190 -> [_ w3234]
          tunnel: [w3217 w3225] -> w3183
          tunnel: w3187 -> [w3217 _]
          tunnel: [w3216 w3224] -> w3184
          tunnel: w3185 -> [w3216 _]
          frame False {
            n1902 = Increment(x=w3223) -> (x+1=w3221:i32)
          }
          frame True {
            w3231 = FALSE ("Start Saving")
            w3236 = 9.0  # File Version
            w3244 = FALSE ("prepend array or string size? (T)")
            w3242 = T29."big-endian, network order" ("byte order (0:big-endian, network order)")
            # "write file headers"
            n1903 = local read "BD 1 Frequency 1 (MHz)"() -> (w3258:dbl)
            n1904 = local read "BD 2 Frequency 1 (MHz)"() -> (w3257:dbl)
            n1905 = local read "BD 1 Frequency 2 (MHz)"() -> (w3256:dbl)
            n1906 = local read "BD 2 Frequency 2 (MHz)"() -> (w3255:dbl)
            n1907 = local read "BD 1 Frequency 3 (MHz)"() -> (w3254:dbl)
            n1908 = local read "BD 2 Frequency 3 (MHz)"() -> (w3253:dbl)
            n1909 = Array Size(array=w3234) -> (size(s)=w3233:i32)
            n1910 = To Double Precision Float(number=w3233) -> (double precision float=w3232:dbl)
            n1911 = local write "Save Calibration"(w3231) -> ()
            n1912 = local write "Start Saving"(w3231) -> ()
            n1913 = Build Array("Save APD Data\nwith Trap Data", "Save Trap Pos. Data") -> (w3228:bool[])
            n1914 = Boolean Array To Number(Boolean array=w3228) -> (number=w3227:u32)
            n1915 = Build Array(w3258, w3257, w3256, w3255, w3254, w3253) -> (w3252:dbl[])
            n1916 = case shown="2" w3262 {
              tunnel: w3261 -> [w3333 w3353 w3369 w3407]
              tunnel: w3232 -> [w3338 w3360 w3389 w3426]
              tunnel: w3259 -> [w3337 w3359 w3388 w3425]
              tunnel: [w3334 w3355 w3380 w3417] -> w3250
              tunnel: [w3325 "Cal sets to save" w3370 w3408] -> w3240
              tunnel: w3252 -> [w3335 w3356 w3382 w3419]
              tunnel: "Save APD Data\nwith Trap Data" -> [w3332 _ w3366 w3405]
              tunnel: [w3332 w3347 w3366 w3405] -> w3237
              tunnel: w3236 -> [w3328 w3348 w3364 w3403]
              tunnel: w3235 -> [w3327 _ _ _]
              tunnel: [w3318 w3347 w3363 w3393] -> w3224
              tunnel: "Save Trap Pos. Data" -> [w3318 _ w3363 w3393]
              tunnel: w3227 -> [w3317 _ w3362 w3392]
              frame 1, Default {
                # "timeseries"
                n1917 = case shown="True" "Profile" {
                  tunnel: [w3341 w3344] -> w3322
                  tunnel: [w3341 w3343] -> w3321
                  tunnel: [w3341 w3342] -> w3320
                  tunnel: [w3341 w3346] -> w3319
                  frame False {
                    w3341 = 0.0 ("f")
                  }
                  frame True {
                    n1918 = local read "Current Position"() -> (w3345:dbl[])
                    n1919 = local read "Y change (mm)"() -> (w3346:dbl)
                    n1920 = call "subVI_explode3array.vi"("Array"=w3345) -> ("x"=w3344:dbl, "y"=w3343:dbl, "z"=w3342:dbl)  [unwired: 12 in]
                  }
                }
                n1921 = local read "Save ave N"() -> (w3340:dbl)
                n1922 = Multiply(x=w3340, y=w3333) -> (x*y=w3339:dbl)
                n1923 = To Double Precision Float(number=w3317) -> (double precision float=w3331:dbl)
                n1924 = Build Array(w3328, w3333, w3339, w3338, w3337, 0.0 ("f")) -> (w3336:dbl[])
                n1925 = Build Array(w3331, w3322, w3321, w3320, w3319) -> (w3329:dbl[])
                n1926 = Select(t=u32 4000000000, s=w3327, f="N sets to save") -> (s? t:f=w3325:u32)
                n1927 = Build Array (concatenate)(w3336, w3335, w3329) -> (w3334:dbl[])
              }
              frame 2 {
                w3350 = 0.0 ("f")
                w3347 = FALSE ("Save APD Data\nwith Trap Data")
                # "calibration"
                n1928 = Boolean To (0,1)(Boolean=w3347) -> (0, 1=w3352:i16)
                n1929 = To Double Precision Float(number=w3352) -> (double precision float=w3351:dbl)
                n1930 = Build Array(w3351, w3350, w3350, w3350, w3350) -> (w3349:dbl[])
                n1931 = Build Array(w3348, w3353, w3353, w3360, w3359, 1.0 ("t")) -> (w3357:dbl[])
                n1932 = Build Array (concatenate)(w3357, w3356, w3349) -> (w3355:dbl[])
                "Calibrating Trap..." <- TRUE ("Calibrating...")
              }
              frame 4 {
                w3367 = 0.0 ("f")
                # "write file header for a trap \nraster scan"
                # "scan dir (x/y = 0/1)"
                # "cycles/step"
                # "n scans (f/b)"
                # "steps"
                # "freq. range"
                # "AOD raster scan"
                n1933 = local read "Number of F/B Scans (AOD)"() -> (w3374:u16)
                n1934 = local read "Cycles/step (AOD)"() -> (w3376:u64)
                n1935 = local read "Scan Range (MHz)"() -> (w3379:dbl)
                n1936 = local read "Scan steps (AOD)"() -> (w3378:u64)
                n1937 = local read "Scan BD"() -> (w3386:bool)
                n1938 = local read "Save ave N"() -> (w3391:dbl)
                n1939 = Boolean To (0,1)(Boolean=w3386) -> (0, 1=w3385:i16)
                n1940 = To Double Precision Float(number=w3374) -> (double precision float=w3373:dbl)
                n1941 = To Double Precision Float(number=w3378) -> (double precision float=w3377:dbl)
                n1942 = To Double Precision Float(number=w3376) -> (double precision float=w3375:dbl)
                n1943 = To Double Precision Float(number=w3385) -> (double precision float=w3384:dbl)
                n1944 = Multiply(x=w3391, y=w3369) -> (x*y=w3390:dbl)
                n1945 = To Double Precision Float(number=w3362) -> (double precision float=w3368:dbl)
                n1946 = Build Array(w3368, w3367, w3367, w3367, w3367) -> (w3365:dbl[])
                n1947 = local read "N sets should be saved"() -> (w3371:dbl)
                n1948 = Build Array(w3384, w3379, w3377, w3375, w3373) -> (w3381:dbl[])
                n1949 = Build Array(w3364, w3369, w3390, w3389, w3388, 2.0 ("t")) -> (w3383:dbl[])
                n1950 = Round Toward +Infinity(x=w3371) -> (ceil(x): smallest int >= x=w3372:dbl)
                n1951 = Build Array (concatenate)(w3383, w3382, w3365, w3381) -> (w3380:dbl[])
                n1952 = To Unsigned Long Integer(number=w3372) -> (unsigned 32bit integer=w3370:u32)
              }
              frame 8 {
                w3400 = 0.0 ("f")
                # "MCL raster scan"
                n1953 = local read "Number of scans (MCL)"() -> (w3395:u64)
                n1954 = local read "Scan lines (y)"() -> (w3394:u64)
                n1955 = local read "2D or 1D Scan"() -> (w3397:bool)
                n1956 = local read "Scan Range (V)\n(of steps)"() -> (w3416:dbl)
                n1957 = local read "Fast Scan Dir"() -> (w3423:bool)
                n1958 = local read "Cycles/step (MCL)"() -> (w3413:u64)
                n1959 = local read "Scan steps (MCL)"() -> (w3415:u64)
                n1960 = Select(t=w3394, s=w3397, f=w3395) -> (s? t:f=w3396:u64)
                n1961 = Boolean To (0,1)(Boolean=w3397) -> (0, 1=w3399:i16)
                n1962 = local read "Save ave N"() -> (w3428:dbl)
                n1963 = local read "Initial X"() -> (w3402:dbl)
                n1964 = local read "Initial Y"() -> (w3401:dbl)
                n1965 = To Double Precision Float(number=w3399) -> (double precision float=w3398:dbl)
                n1966 = Boolean To (0,1)(Boolean=w3423) -> (0, 1=w3422:i16)
                n1967 = To Double Precision Float(number=w3396) -> (double precision float=w3411:dbl)
                n1968 = To Double Precision Float(number=w3415) -> (double precision float=w3414:dbl)
                n1969 = To Double Precision Float(number=w3413) -> (double precision float=w3412:dbl)
                n1970 = To Double Precision Float(number=w3422) -> (double precision float=w3421:dbl)
                n1971 = Multiply(x=w3428, y=w3407) -> (x*y=w3427:dbl)
                n1972 = To Double Precision Float(number=w3392) -> (double precision float=w3406:dbl)
                n1973 = local read "N sets should be saved (MCL)"() -> (w3409:dbl)
                n1974 = Build Array(w3406, w3398, w3400, w3400, w3400) -> (w3404:dbl[])
                n1975 = Build Array(w3421, w3416, w3414, w3412, w3411, w3402, w3401) -> (w3418:dbl[])
                n1976 = Build Array(w3403, w3407, w3427, w3426, w3425, 3.0 ("t")) -> (w3420:dbl[])
                n1977 = Round Toward +Infinity(x=w3409) -> (ceil(x): smallest int >= x=w3410:dbl)
                n1978 = Build Array (concatenate)(w3420, w3419, w3404, w3418) -> (w3417:dbl[])
                n1979 = To Unsigned Long Integer(number=w3410) -> (unsigned 32bit integer=w3408:u32)
              }
            }
            n1980 = local read "Index"() -> (w3267:dbl)
            n1981 = call "Create new save file.vi"("Insert"="", "Ext"=".dat", "Index In"=w3267) -> ("Path Out"=w3226:path, "Index Out"=w3239:dbl)
            n1982 = local write "Save file name"(w3226) -> ()
            n1983 = local write "Index"(w3239) -> ()
